vi "Int16Array Destroy.vi"(8 "error in (no error)":errorcluster, 11 "Int16Array DVR in":refnum<data-value>) -> (0 "error out":errorcluster)   [LabVIEW 2012, in "MDSplus.lvlib"]
uses:
  <vilib>/MDSplus/Library/MDSplus.lvlib
  <vilib>/MDSplus/Classes/Data_Class/Array_Class/Int16Array_Class/Int16Array.lvclass
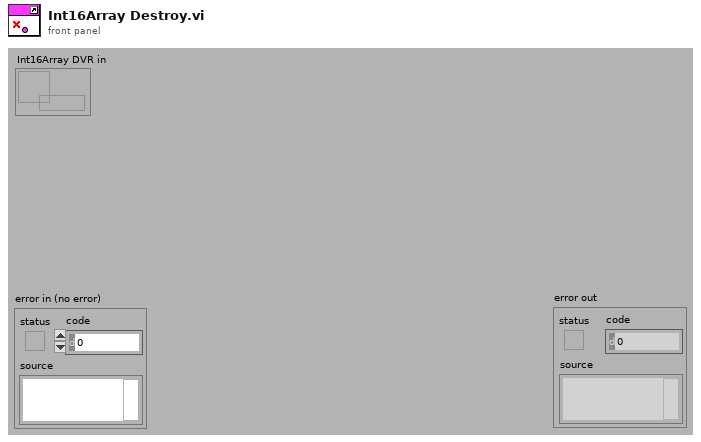
[diagram p1: front panel]
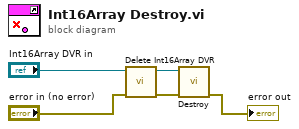
[diagram p0: block diagram]
diagram:
  n1 = call <vilib>:"Delete Int16Array DVR.vi"("error in (no error)"="error in (no error)", "Int16Array DVR in"="Int16Array DVR in") -> ("error out"=w2:errorcluster, "Int16Array out"=w3:refnum<class "Int16Array.lvclass">)  [unwired: 8 in]
  n2 = call-dynamic "Destroy.vi"("error in (no error)"=w2, "Int16Array in"=w3) -> ("error out"=→"error out":errorcluster)  [unwired: 9 in]
